vi "Untitled 2.vi"() -> ()   [LabVIEW 2015]
uses:
  BoardDisplay.lvclass
  TronviewGame/GameRecorder/GameRecorder.lvclass
panel:
  in  "Game string":string="p1;p2;16,16,0,0,0,0,0,0,0,0,0,0,0,0,0,0,0,0,0,0,0,0,0,0,0,0,0,0,0,0,0,0,0,0,0,0,2,0,0,0,0,0,0,0,0,0,0,0,0,0,0,0,0,0,0,0,0,0,0,0,0,0,0,0,0,0,0,0,0,0,0,0,0,0,0,0,0,0,0,0,0,0,0,0,0,0,0,0,0,0,0,0,0,0,0,0,0,0,0,0,0,0,0,0,0,0,0,0,0,0,0,0,0,0,0,0,0,0,0,0,0,0,0,0,0,0,0,0,0,0,0,0,0,0,0,0,0,0,0,0,0,0,0,0,0,0,0,0,0,0,0,0,0,0,0,0,0,0,0,0,0,0,0,0,0,0,0,0,0,0,0,0,0,0,0,0,0,0,0,0,0,0,0,0,0,0,0,0,0,0,0,0,0,0,0,0,0,0,0,0,0,0,0,0,0,0,0,0,0,0,0,0,0,0,0,0,0,0,0,0,0,0,0,0,0,0,0,0,0,0,0,0,0,0,0,0,0,0,0,0,3,0,0,0,0,0,0,0,0,0,0,0,0,0,0,0,0,0;S,S,S,E,S,W,S,W,N,W,S,S,E,E,S,S,E,N,E,N,E,S,E,S,S,S,E,E,S,W,W,W,W,N,W,W,W,S,W,N,N,E,E,E,E,E,S,S;S,E,N,N,W,W,S,S,W,W,W,W,W,W,W,W,W,W,W,W,W,N,E,E,E,E,E,E,E,E,E,E,E,E,N,W,W,W,N,E,E,E,E,E,E,N,W,W\r\n"
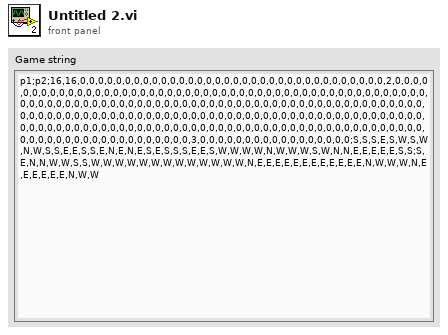
[diagram p1: front panel]
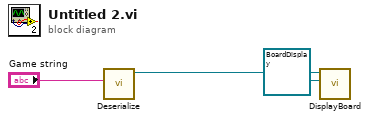
[diagram p0: block diagram]
diagram:
  n1 = call "Deserialize.vi"("String"="Game string") -> ("GameRecorder out"=w2:refnum<class "GameRecorder.lvclass">)  [unwired: 9 in, 1 out]
  n2 = call "DisplayBoard.vi"("GameRecorder"=w2, "BoardDisplay in"=refnum<class "BoardDisplay.lvclass"> refnum) -> ()  [unwired: 5 in, 5 out]
